vi "Configure Trigger Polarity.vi"(7 "Trigger Polarity Positive (T)":bool=TRUE, 8 "error in (no error)":errorcluster, 11 "VISA resource name":refnum<visa-resource-name>) -> (0 "error out":errorcluster, 3 "VISA resource name out":refnum<visa-resource-name>)   [LabVIEW 2020, in "QuPMXdriver.lvlib"]
doc: "Configures trigger polarity to postive or negative."
uses:
  QuPMXdriver.lvlib
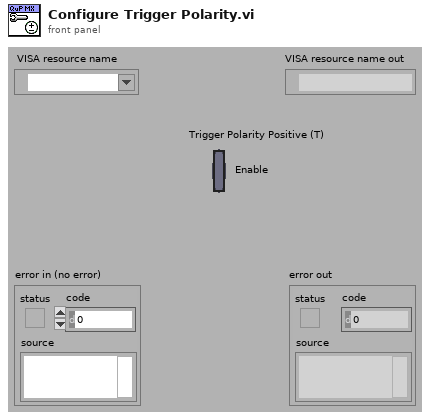
[diagram p1: front panel]
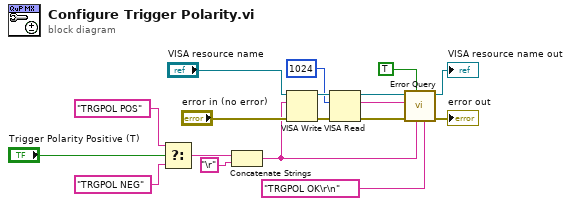
[diagram p0: block diagram]
diagram:
  n1 = Select(t="TRGPOL POS" ("write buffer"), s="Trigger Polarity Positive (T)", f="TRGPOL NEG" ("write buffer")) -> (s? t:f=w12:string)
  n2 = Concatenate Strings(w12, "\r") -> (w6:string)
  n3 = VISA Write(VISA resource name="VISA resource name", write buffer=w6, error in (no error)="error in (no error)") -> (VISA resource name out=w9:refnum<visa-resource-name>, error out=w1:errorcluster)  [unwired: 1 out]
  n4 = VISA Read(VISA resource name=w9, byte count=u32 1024, error in (no error)=w1) -> (VISA resource name out=w8:refnum<visa-resource-name>, read buffer=w5:string, error out=w4:errorcluster)  [unwired: 1 out]
  n5 = call "Error Query.vi"("Expected read buffer"="TRGPOL OK\r\n" ("write buffer"), "Last command"=w6, "Ignore empty sequence? (T)"=TRUE, "error in (no error)"=w4, "Read buffer"=w5, "VISA resource name"=w8) -> ("error out"=→"error out":errorcluster, "VISA resource name out"=→"VISA resource name out":refnum<visa-resource-name>)  [unwired: 4 in]
